vi "Andor Get One Frame - subvi.vi"(8 "error in":errorcluster, 10 "New Image":T1, 11 "Image Size":T2 {"V Bin" min=0.0; "H Bin" min=0.0 step=1.0}) -> (0 "error out":errorcluster, 2 "Image Out":T1)   [LabVIEW 2014]
uses:
  <vilib>/vision/Image Controls.llb/IMAQ Image.ctl
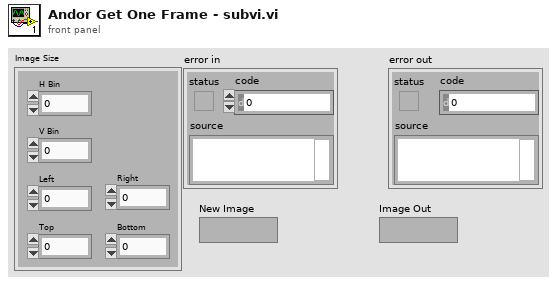
[diagram p1: front panel]
types:
  T1 = typedef "IMAQ Image.ctl" = refnum<image>
  T2 = cluster{"H Bin":dbl, "V Bin":dbl, "Left":dbl, "Right":dbl, "Top":dbl, "Bottom":dbl}
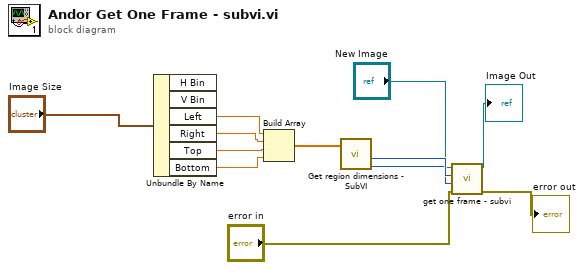
[diagram p0: block diagram]
diagram:
  n1 = Unbundle By Name("Image Size") -> ("Left"=w11:dbl, "Right"=w10:dbl, "Top"=w9:dbl, "Bottom"=w8:dbl)  [unwired: 2 out]
  n2 = Build Array(w11, w10, w9, w8) -> (w7:dbl[])
  n3 = call "Get region dimensions - SubVI.vi"("x1y1x2y2"=w7) -> ("y size"=w5:u16, "x size"=w6:u16)  [unwired: 7 in, 2 out]
  n4 = call "get one frame - subvi.vi"("error in"="error in", "Image Height"=w5, "Image Width"=w6, "Image In"="New Image") -> ("error out"=→"error out":errorcluster, "Image Out"=→"Image Out":T1)  [unwired: 6 in]
